vi "programmatic FTP file transfer.vi"() -> ()   [LabVIEW 2017, in "labview-standard-library.lvlib"]
uses:
  labview-standard-library.lvlib
  <vilib>/FTP/NI_FTP.lvlib
panel:
  in  "IP address of remote RT target":string
  in  "path to directory (on local host)where you want files to be copied":path
  in  "path to directory (on RT target) from which you want to copy files":string
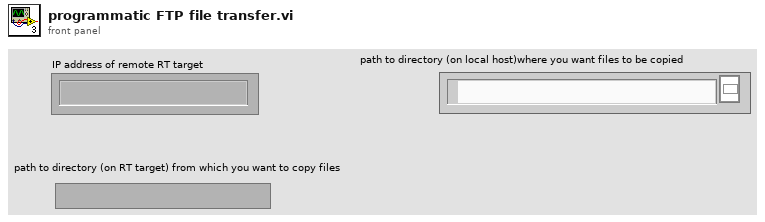
[diagram p1: front panel]
types:
  T1 = typedef "NI_FTP.lvlib/FTP Session.ctl" = refnum<k5>
  T2 = typedef "NI_FTP.lvlib/FTP File Info.ctl" = cluster{"type":enum16{"unknown", "file", "dir", "link"}, "permissions":string, "owner":string, "group":string, "size":i32, "date":string, "name":string, "link name":string}
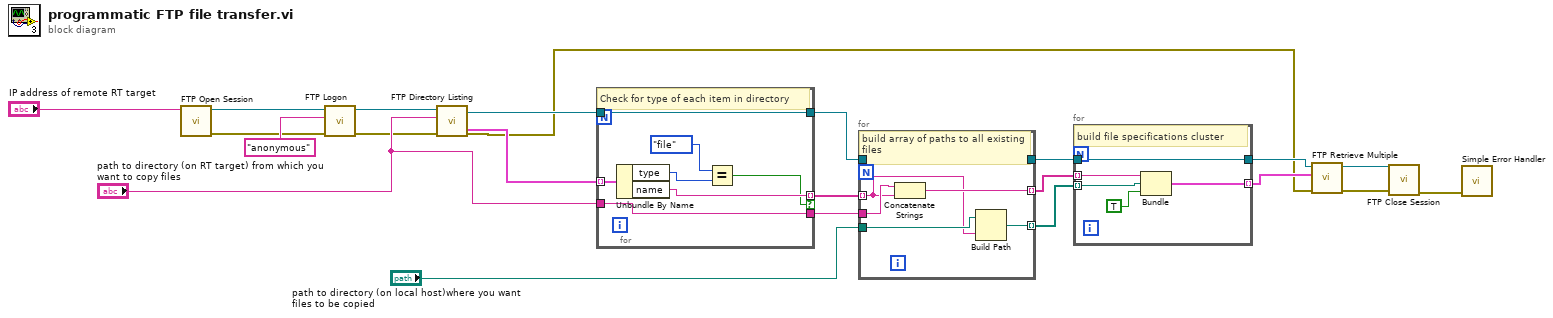
[diagram p0: block diagram]
diagram:
  n1 = call <vilib>:"FTP Open Session.vi"("address"="IP address of remote RT target") -> ("error out"=w4:errorcluster, "ftp session"=w22:T1)  [unwired: 7 in, 2 out]
  n2 = call <vilib>:"FTP Logon.vi"("error in (no error)"=w4, "user"="anonymous", "ftp session"=w22) -> ("error out"=w3:errorcluster, "ftp session out"=w21:T1)  [unwired: 5 in, 2 out]
  n3 = call <vilib>:"FTP Directory Listing.vi"("error in (no error)"=w3, "directory path"="path to directory (on RT target) from which you want to copy files", "ftp session"=w21) -> ("error out"=w2:errorcluster, "ftp session out"=w19:T1, "dir list"=w20:T2[])  [unwired: 4 in, 2 out]
  n4 = for {
    tunnel: w20 -> [w29] mode=indexing
    tunnel: [w28] -> w8
    tunnel: w19 -> [w28]
    tunnel: [w25] -> w17 mode=indexing if=w24
    tunnel: [w23] -> w16
    tunnel: "path to directory (on RT target) from which you want to copy files" -> [w23]
    # "Check for type of each item in directory"
    n5 = Unbundle By Name(w29) -> ("type"=w27:enum16{"unknown", "file", "dir", "link"}, "name"=w25:string)
    n6 = Equal?(x=enum16{"unknown", "file", "dir", "link"}."file", y=w27) -> (x = y?=w24:bool)
  }
  n7 = for {
    tunnel: w17 -> [w30] mode=indexing
    tunnel: w16 -> [w31]
    tunnel: [w35] -> w15 mode=indexing
    tunnel: "path to directory (on local host)where you want files to be copied" -> [w34]
    tunnel: [w33] -> w13 mode=indexing
    tunnel: [w32] -> w9
    tunnel: w8 -> [w32]
    # "build array of paths to all existing files"
    n8 = Concatenate Strings(w31, w30) -> (w35:string)
    n9 = Build Path(base path=w34, name or relative path=w30) -> (appended path=w33:path)
  }
  n10 = for {
    tunnel: w15 -> [w40] mode=indexing
    tunnel: w13 -> [w39] mode=indexing
    tunnel: [w37] -> w12 mode=indexing
    tunnel: [w36] -> w10
    tunnel: w9 -> [w36]
    # "build file specifications cluster"
    n11 = Bundle(w40, "appended path"=w39, TRUE) -> (w37:cluster{string, "appended path":path, bool})  [unwired: 1 in]
  }
  n12 = call <vilib>:"FTP Retrieve Multiple.vi"("error in (no error)"=w2, "file specifications"=w12, "ftp session"=w10) -> ("error out"=w5:errorcluster, "ftp session out"=w6:T1)  [unwired: 5 in, 2 out]
  n13 = call <vilib>:"FTP Close Session.vi"("error in (no error)"=w5, "ftp session"=w6) -> ("error out"=w1:errorcluster)  [unwired: 6 in, 3 out]
  n14 = call <vilib>:"Simple Error Handler.vi"("error in (no error)"=w1) -> ()  [unwired: 4 in, 5 out]
